vi "Get Request Type.vi"(8 "error in (no error)":errorcluster, 11 "SetCurrentProgramScene in":refnum<class "SetCurrentProgramScene.lvclass">) -> (0 "error out":errorcluster, 2 "Request Type":string, 3 "SetCurrentProgramScene out":refnum<class "SetCurrentProgramScene.lvclass">)   [LabVIEW 2022 SP3, in "obs-websocket-lv.lvlib" / "SetCurrentProgramScene.lvclass"]
uses:
  SetCurrentProgramScene.lvclass
  SetCurrentProgramScene.lvclass/SetCurrentProgramScene.ctl
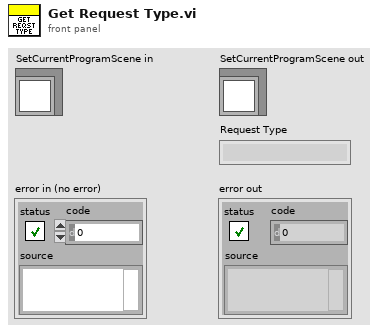
[diagram p1: front panel]
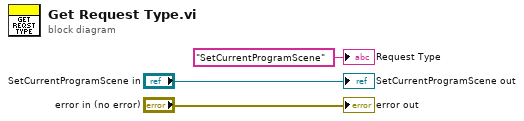
[diagram p0: block diagram]
diagram:
  "error out" <- "error in (no error)"
  "SetCurrentProgramScene out" <- "SetCurrentProgramScene in"
  "Request Type" <- "SetCurrentProgramScene" ("Request Type")
